vi "MCDC VISA Low Level COMs.vi"(7 "Action":T1=enum."Close Session", 8 "error in (no error)":errorcluster, 10 "Send Message":string, 11 "VISA resource name":refnum<visa-resource-name>) -> (0 "error out":errorcluster, 1 "Value":dbl, 2 "Message":string, 5 "Active?":bool)   [LabVIEW 2018]
uses:
  General/Controls/Low Level Com Actions.ctl
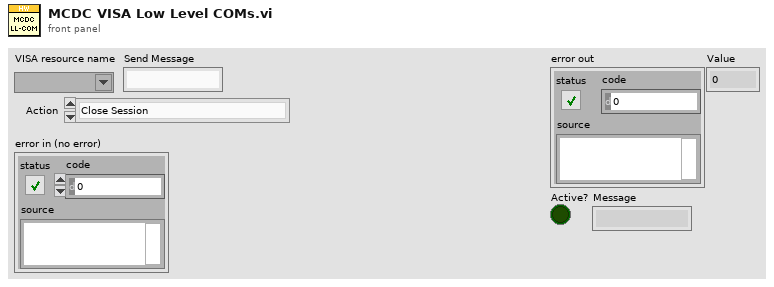
[diagram p1: front panel]
types:
  T1 = typedef "Low Level Com Actions.ctl" = enum16{"Open Session", "Close Session", "Send Command", "Query Command"}
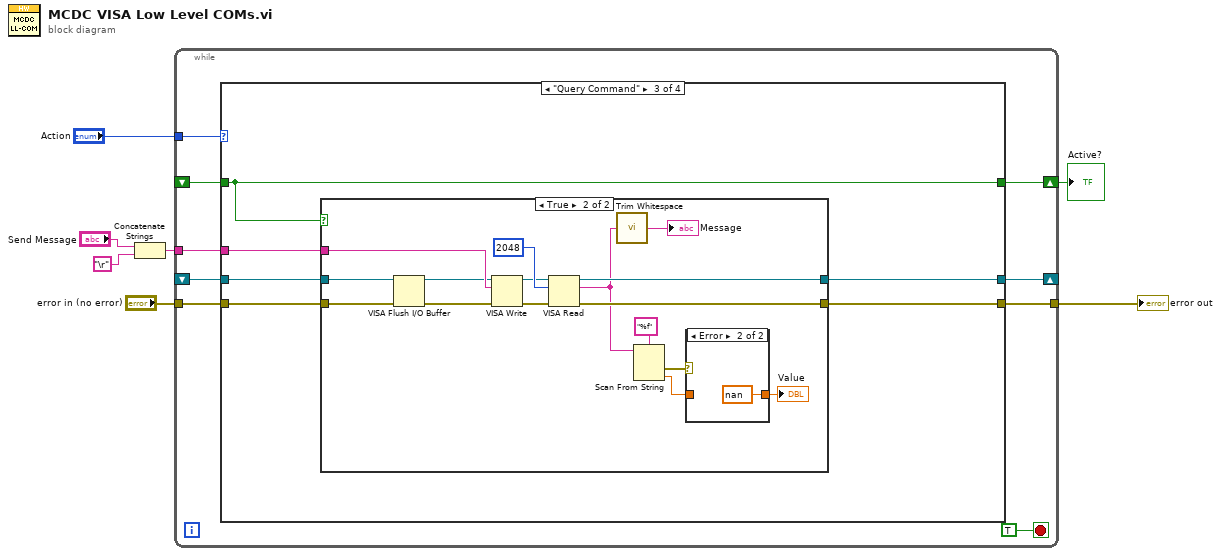
[diagram p0: block diagram]
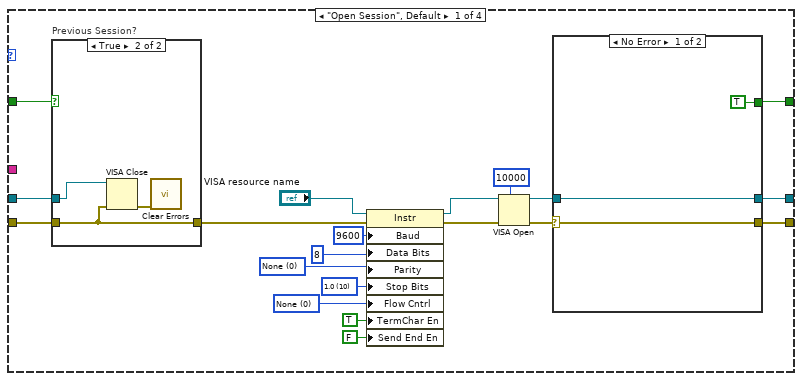
[diagram p2: hidden frame]
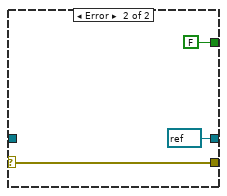
[diagram p4: hidden frame]
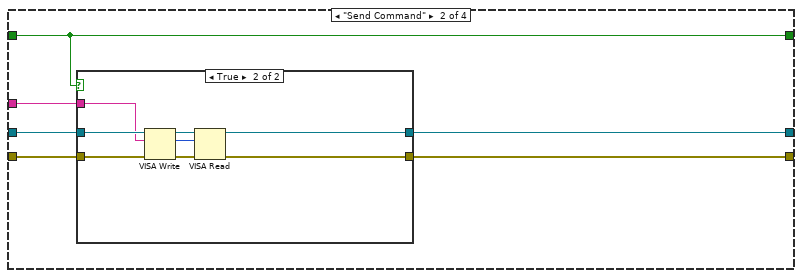
[diagram p5: hidden frame]
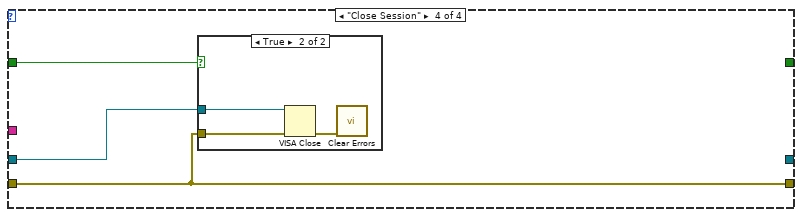
[diagram p9: hidden frame]
diagram:
  n1 = Concatenate Strings("Send Message", "\r") -> (w1:string)
  n2 = while {
    tunnel: "Action" -> [w16]
    tunnel: "error in (no error)" -> [w15]
    shift-right: [w13] -> _
    shift-left: _ -> [w12]
    tunnel: [w11] -> w5
    shift-right: [w10] -> w4
    shift-left: _ -> [w9]
    tunnel: w1 -> [w8]
    stop <- TRUE stop-if-true
    n3 = case shown="\"Query Command\"" w16 {
      tunnel: w15 -> [w30 w52 w68 w90]
      tunnel: [w33 w49 w65 _] -> w13
      tunnel: w12 -> [w29 w51 w67 w91]
      tunnel: [w32 w50 w66 w90] -> w11
      tunnel: [w31 w48 w64 _] -> w10
      tunnel: w9 -> [w27 w48 w64 w89]
      tunnel: w8 -> [_ w47 w63 _]
      frame "Open Session", Default {
        w17 = u16 0 items=["None", "XON/XOFF", "RTS/CTS", "XON/XOFF & RTS/CTS", "DTR/DSR", "XON/XOFF & DTR/DSR"] ("Serial Settings:Flow Control")
        w18 = u16 10 items=["1.0"=10, "1.5"=15, "2.0"=20] ("Serial Settings:Stop Bits")
        w19 = u16 0 items=["None", "Odd", "Even", "Mark", "Space"] ("Serial Settings:Parity")
        n4 = case "Previous Session?" shown="True" w27 {
          tunnel: w30 -> [w37 w38]
          tunnel: w29 -> [_ w40]
          tunnel: [w37 w38] -> w28
          frame False {
          }
          frame True {
            n5 = VISA Close(VISA resource name=w40, error in (no error)=w38) -> (error out=w39:errorcluster)
            n6 = call <vilib>:"Clear Errors.vi"("error in (no error)"=w39) -> ()  [unwired: 5 in, 2 out]
          }
        }
        n7 = property class="Instr"(reference="VISA resource name", error in=w28, "Baud"=u32 9600 ("Serial Settings:Baud Rate"), "Data Bits"=u16 8 ("Serial Settings:Data Bits"), "Parity"=w19, "Stop Bits"=w18, "Flow Cntrl"=w17, "TermChar En"=TRUE ("Message Based Settings:Termination Character Enable"), "Send End En"=FALSE ("Message Based Settings:Send End Enable")) -> (reference out=w24:refnum<visa-resource-name>, error out=w26:errorcluster)
        n8 = VISA Open(timeout (0)=u32 10000 ("VISA Open timeout (0)"), error in (no error)=w26, VISA resource name=w24) -> (VISA resource name=w34:refnum<visa-resource-name>, error out=w35:errorcluster)  [unwired: 2 in]
        n9 = case shown="No Error" w35 {
          selector: w35 -> [w42 w45]
          tunnel: w34 -> [w43 _]
          tunnel: [w43 refnum<visa-resource-name> refnum ("VISA resource name")] -> w33
          tunnel: [w42 w45] -> w32
          tunnel: [TRUE FALSE] -> w31
          frame No Error {
          }
          frame Error {
          }
        }
      }
      frame "Send Command" {
        n10 = case shown="True" w48 {
          tunnel: w52 -> [w54 w62]
          tunnel: w51 -> [w53 w61]
          tunnel: [w54 w58] -> w50
          tunnel: [w53 w55] -> w49
          tunnel: w47 -> [_ w59]
          frame False {
          }
          frame True {
            n11 = VISA Write(VISA resource name=w61, write buffer=w59, error in (no error)=w62) -> (VISA resource name out=w57:refnum<visa-resource-name>, return count=w56:u32, error out=w60:errorcluster)
            n12 = VISA Read(VISA resource name=w57, byte count=w56, error in (no error)=w60) -> (VISA resource name out=w55:refnum<visa-resource-name>, error out=w58:errorcluster)  [unwired: 2 out]
          }
        }
      }
      frame "Query Command" {
        n13 = case shown="True" w64 {
          tunnel: w68 -> [w69 w77]
          tunnel: w67 -> [w70 w71]
          tunnel: [w69 w86] -> w66
          tunnel: [w70 w85] -> w65
          tunnel: w63 -> [_ w75]
          frame False {
          }
          frame True {
            n14 = VISA Flush I/O Buffer(VISA resource name=w71, error in (no error)=w77) -> (VISA resource name out=w72:refnum<visa-resource-name>, error out=w73:errorcluster)  [unwired: 1 in]
            n15 = VISA Write(VISA resource name=w72, write buffer=w75, error in (no error)=w73) -> (VISA resource name out=w74:refnum<visa-resource-name>, error out=w76:errorcluster)  [unwired: 1 out]
            n16 = VISA Read(VISA resource name=w74, byte count=u32 2048, error in (no error)=w76) -> (VISA resource name out=w85:refnum<visa-resource-name>, read buffer=w80:string, error out=w86:errorcluster)  [unwired: 1 out]
            n17 = call <vilib>:"Trim Whitespace.vi"("string"=w80) -> ("trimmed string"=→"Message":string)  [unwired: 1 in]
            n18 = Scan From String(format string="%f", input string=w80) -> (error out=w81:errorcluster, output 1=w79:dbl)  [unwired: 3 in, 2 out]
            n19 = case shown="Error" w81 {
              tunnel: w79 -> [w87 _]
              tunnel: [w87 nan] -> w78
              frame No Error {
              }
              frame Error {
              }
            }
            "Value" <- w78
          }
        }
      }
      frame "Close Session" {
        n20 = case shown="True" w89 {
          tunnel: w91 -> [_ w94]
          tunnel: w90 -> [_ w93]
          frame False {
          }
          frame True {
            n21 = VISA Close(VISA resource name=w94, error in (no error)=w93) -> (error out=w92:errorcluster)
            n22 = call <vilib>:"Clear Errors.vi"("error in (no error)"=w92) -> ()  [unwired: 5 in, 2 out]
          }
        }
      }
    }
  }
  "error out" <- w5
  "Active?" <- w4
